vi "Acquire.vi"(0 "Acquisition Unit in (0)":i32, 1 "Replay settings":T19={"Sampling Rate"=0.0, "Samples in replay"=0, "Replay Start Time"=1000.0, "Replay Stop Time"=0.003} {"Replay Stop Time" format="%.3p"; "Replay Start Time" format="%.3p"}, 5 "Acquire Definition":T3={"Acquire Mode"=enum."stop", "Acquisition mode"=enum."Sampled", "Acquirer"=enum."Cleverscope", "Transfer Chans"=enum."Chan A+B", "A max scale"=5.0, "A min scale"=-5.0, "B max scale"=5.0, "B min scale"=-5.0, "A Probe"=enum."x1", "B Probe"=enum."x1", "A Coupling"=enum."DC", "B Coupling"=enum."DC", "A Bandwidth"=1, "B Bandwidth"=1, "Trigger Source"=enum."Chan A", "Trigger Amplitude"=0.0, "A Trigger Amplitude"=0.0, "B Trigger Amplitude"=0.0, "Trigger Filter"=enum."None", "Trig Slope"=FALSE, "Trigger Holdoff"=0.0, "Dig Pattern Rqd"=FALSE, "Dig Pattern"=0, "Ext Trig Threshold"=0.0, "Dig Input Threshold"=0.0, "Start Time"=-0.003, "Stop Time"=0.003, "Pre Trig Time"=0.003, "Port"=enum."Port 1", "Num divisions"=6, "Num seq frames"=1, "Num Buffers"=2, "Sig Gen Freq"=1000.0, "Sig Gen Amp"=1.0, "Sig Gen Offset"=0.0, "Sig Gen Waveform"=enum."sine", "Sig Gen Sweep"=enum."Log", "Sig Gen Func"=enum."Standard", "Sig Gen Freq 2"=1000.0, "Sig Gen Phase"=180.0, "Trig 2 Function"=enum."None", "Min Trigger Period"=1e-08, "Max trigger Period"=0.0001, "Trigger count"=1, "Trig 2 Slope"=FALSE, "Trig 2 Source Chan"=enum."Chan A", "Trig 2 Level"=0.0, "Dig Pattern 2 Rqd"=FALSE, "Dig Pattern 2"=0, "Trigger 2 Source"=enum."Trigger 1 inverted", "Waveform Averages"=0, "Value changed"=0, "Freq Span"=0.0, "Freq Res"=0.0, "Duration"=0.0, "Resolution"=0.0, "Link Port"=enum."Debug", "Ext Sample Clock"=FALSE, "F Spare 2"=FALSE, "F Spare 3"=FALSE, "F Spare 4"=FALSE, "Sampler Resolution"=enum."10 bit", "Intf Source"=enum."USB", "Update Rate"=enum."20 Frame/sec", "Transfer Size"=enum."Normal", "Sig Gen Freq Step"=0.0, "TCP Adr"=0, "TCP port"=0, "CAU Ser Num Hi"=0, "CAU Ser Num Lo"=0, "Function Number"=0.0, "Function Parameter"=0.0, "Function Result"=0.0, "Link Start"=0, "Link Timebase"=0, "Link Timer"=0, "Link Setup"=0, "Spare 1"=0.0, "Spare 2"=0.0, "Spare 3"=0.0, "Spare 4"=0.0} {"Function Result" format="%#.6p"; "Function Parameter" format="%#.6p"; "Function Number" format="%#.6p"; "TCP Adr" format="%08x"; "Sig Gen Freq Step" format="%.2f"; "Sig Gen Phase" format="%.2f"; "Sig Gen Freq 2" format="%.2f"; "Resolution" format="%#.6p"; "Duration" format="%#.6p"; "Freq Res" format="%#.6p"; "Freq Span" format="%#.6p"; "Dig Pattern 2" format="%.0x"; "Trig 2 Level" step=0.001 format="%#.6p"; "Trigger count" step=1; "Max trigger Period" min=1e-08 max=42.9 step=0.01 format="%#.6p"; "Min Trigger Period" min=1e-08 max=42.9 step=0.01 format="%#_6p"; "Sig Gen Offset" format="%.2f"; "Sig Gen Amp" format="%.2f"; "Sig Gen Freq" format="%.2f"; "B Trigger Amplitude" format="%.1p"; "A Trigger Amplitude" format="%.1p"; "B Bandwidth" format="%x"; "A Bandwidth" format="%x"; "B min scale" format="%.2p"; "B max scale" format="%.2p"; "A min scale" format="%.2p"; "A max scale" format="%.2p"; "Trigger Holdoff" format="%.1p"; "Dig Input Threshold" format="%.2f"; "Ext Trig Threshold" format="%.2f"; "Dig Pattern" format="%.0x"; "Pre Trig Time" format="%.3p"; "Start Time" format="%.2p"; "Trigger Amplitude" format="%.1p"; "Stop Time" format="%.2p"}, 11 "error in (no error)":errorcluster, 12 "Stop Refnum":refnum<vi>) -> (3 "T0dt":T2={"T0"=0.0, "dt"=1.0, "n"=0} {"dt" format="%.3p"; "T0" format="%.3p"}, 4 "Acquisition Unit out":i32, 6 "Acquire Defn Out":T3={"Acquire Mode"=enum."stop", "Acquisition mode"=enum."Sampled", "Acquirer"=enum."Cleverscope", "Transfer Chans"=enum."Chan A+B", "A max scale"=5.0, "A min scale"=-5.0, "B max scale"=5.0, "B min scale"=-5.0, "A Probe"=enum."x1", "B Probe"=enum."x1", "A Coupling"=enum."DC", "B Coupling"=enum."DC", "A Bandwidth"=1, "B Bandwidth"=1, "Trigger Source"=enum."Chan A", "Trigger Amplitude"=0.0, "A Trigger Amplitude"=0.0, "B Trigger Amplitude"=0.0, "Trigger Filter"=enum."None", "Trig Slope"=FALSE, "Trigger Holdoff"=0.0, "Dig Pattern Rqd"=FALSE, "Dig Pattern"=0, "Ext Trig Threshold"=0.0, "Dig Input Threshold"=0.0, "Start Time"=-0.003, "Stop Time"=0.003, "Pre Trig Time"=0.003, "Port"=enum."Port 1", "Num divisions"=6, "Num seq frames"=1, "Num Buffers"=2, "Sig Gen Freq"=1000.0, "Sig Gen Amp"=1.0, "Sig Gen Offset"=0.0, "Sig Gen Waveform"=enum."sine", "Sig Gen Sweep"=enum."Log", "Sig Gen Func"=enum."Standard", "Sig Gen Freq 2"=1000.0, "Sig Gen Phase"=180.0, "Trig 2 Function"=enum."None", "Min Trigger Period"=1e-08, "Max trigger Period"=0.0001, "Trigger count"=1, "Trig 2 Slope"=FALSE, "Trig 2 Source Chan"=enum."Chan A", "Trig 2 Level"=0.0, "Dig Pattern 2 Rqd"=FALSE, "Dig Pattern 2"=0, "Trigger 2 Source"=enum."Trigger 1 inverted", "Waveform Averages"=0, "Value changed"=0, "Freq Span"=0.0, "Freq Res"=0.0, "Duration"=0.0, "Resolution"=0.0, "Link Port"=enum."Debug", "Ext Sample Clock"=FALSE, "F Spare 2"=FALSE, "F Spare 3"=FALSE, "F Spare 4"=FALSE, "Sampler Resolution"=enum."10 bit", "Intf Source"=enum."USB", "Update Rate"=enum."20 Frame/sec", "Transfer Size"=enum."Normal", "Sig Gen Freq Step"=0.0, "TCP Adr"=0, "TCP port"=0, "CAU Ser Num Hi"=0, "CAU Ser Num Lo"=0, "Function Number"=0.0, "Function Parameter"=0.0, "Function Result"=0.0, "Link Start"=0, "Link Timebase"=0, "Link Timer"=0, "Link Setup"=0, "Spare 1"=0.0, "Spare 2"=0.0, "Spare 3"=0.0, "Spare 4"=0.0} {"Function Result" format="%#.6p"; "Function Parameter" format="%#.6p"; "Function Number" format="%#.6p"; "TCP Adr" format="%08x"; "Sig Gen Freq Step" format="%.2f"; "Sig Gen Phase" format="%.2f"; "Sig Gen Freq 2" format="%.2f"; "Resolution" format="%#.6p"; "Duration" format="%#.6p"; "Freq Res" format="%#.6p"; "Freq Span" format="%#.6p"; "Dig Pattern 2" format="%.0x"; "Trig 2 Level" step=0.001 format="%#.6p"; "Trigger count" step=1; "Max trigger Period" min=1e-08 max=42.9 step=0.01 format="%#.6p"; "Min Trigger Period" min=1e-08 max=42.9 step=0.01 format="%#_6p"; "Sig Gen Offset" format="%.2f"; "Sig Gen Amp" format="%.2f"; "Sig Gen Freq" format="%.2f"; "B Trigger Amplitude" format="%.1p"; "A Trigger Amplitude" format="%.1p"; "B Bandwidth" format="%x"; "A Bandwidth" format="%x"; "B min scale" format="%.2p"; "B max scale" format="%.2p"; "A min scale" format="%.2p"; "A max scale" format="%.2p"; "Trigger Holdoff" format="%.1p"; "Dig Input Threshold" format="%.2f"; "Ext Trig Threshold" format="%.2f"; "Dig Pattern" format="%.0x"; "Pre Trig Time" format="%.3p"; "Start Time" format="%.2p"; "Trigger Amplitude" format="%.1p"; "Stop Time" format="%.2p"}, 8 "Chan AB Data":cluster{"Chan A Data":T1[], "Chan B Data":T1[]} {"Chan A Data" format="%_6p"; "Chan B Data" format="%_6p"}, 14 "Waveform":waveform(sgl)[](array[waveform]), 15 "error out":errorcluster)   [LabVIEW 2009]
uses:
  libraries/Cscope control driver.llb/Acquire Event type.ctl
  libraries/Cscope control driver.llb/Acquire capture type.ctl
  libraries/Cscope control driver.llb/Acquire capture method.ctl
  libraries/Cscope control driver.llb/Acquirer type.ctl
  libraries/Cscope control driver.llb/Input Range.ctl
  libraries/Cscope control driver.llb/Input Coupling.ctl
  libraries/Cscope control driver.llb/Input Bandwidth.ctl
  libraries/Cscope control driver.llb/USB channel.ctl
  libraries/Cscope control driver.llb/Trigger Filter.ctl
  libraries/Cscope control driver.llb/Cscope waveform type.ctl
  libraries/Cscope control driver.llb/Trigger Period.ctl
  libraries/Cscope control driver.llb/Trigger channel.ctl
  libraries/Cscope control driver.llb/Link port types.ctl
  libraries/Cscope control driver.llb/Acquirer resolution.ctl
  libraries/Cscope control driver.llb/Intf source.ctl
  libraries/Cscope control driver.llb/Acquire transfer size.ctl
  typedefs/Cscope/ReplaySettings.ctl
  libraries/Cscope control driver.llb/QSig_T0dt.ctl
  libraries/Cscope control driver.llb/Cscope real.ctl
  libraries/Cscope control driver.llb/Cscope control command type.ctl
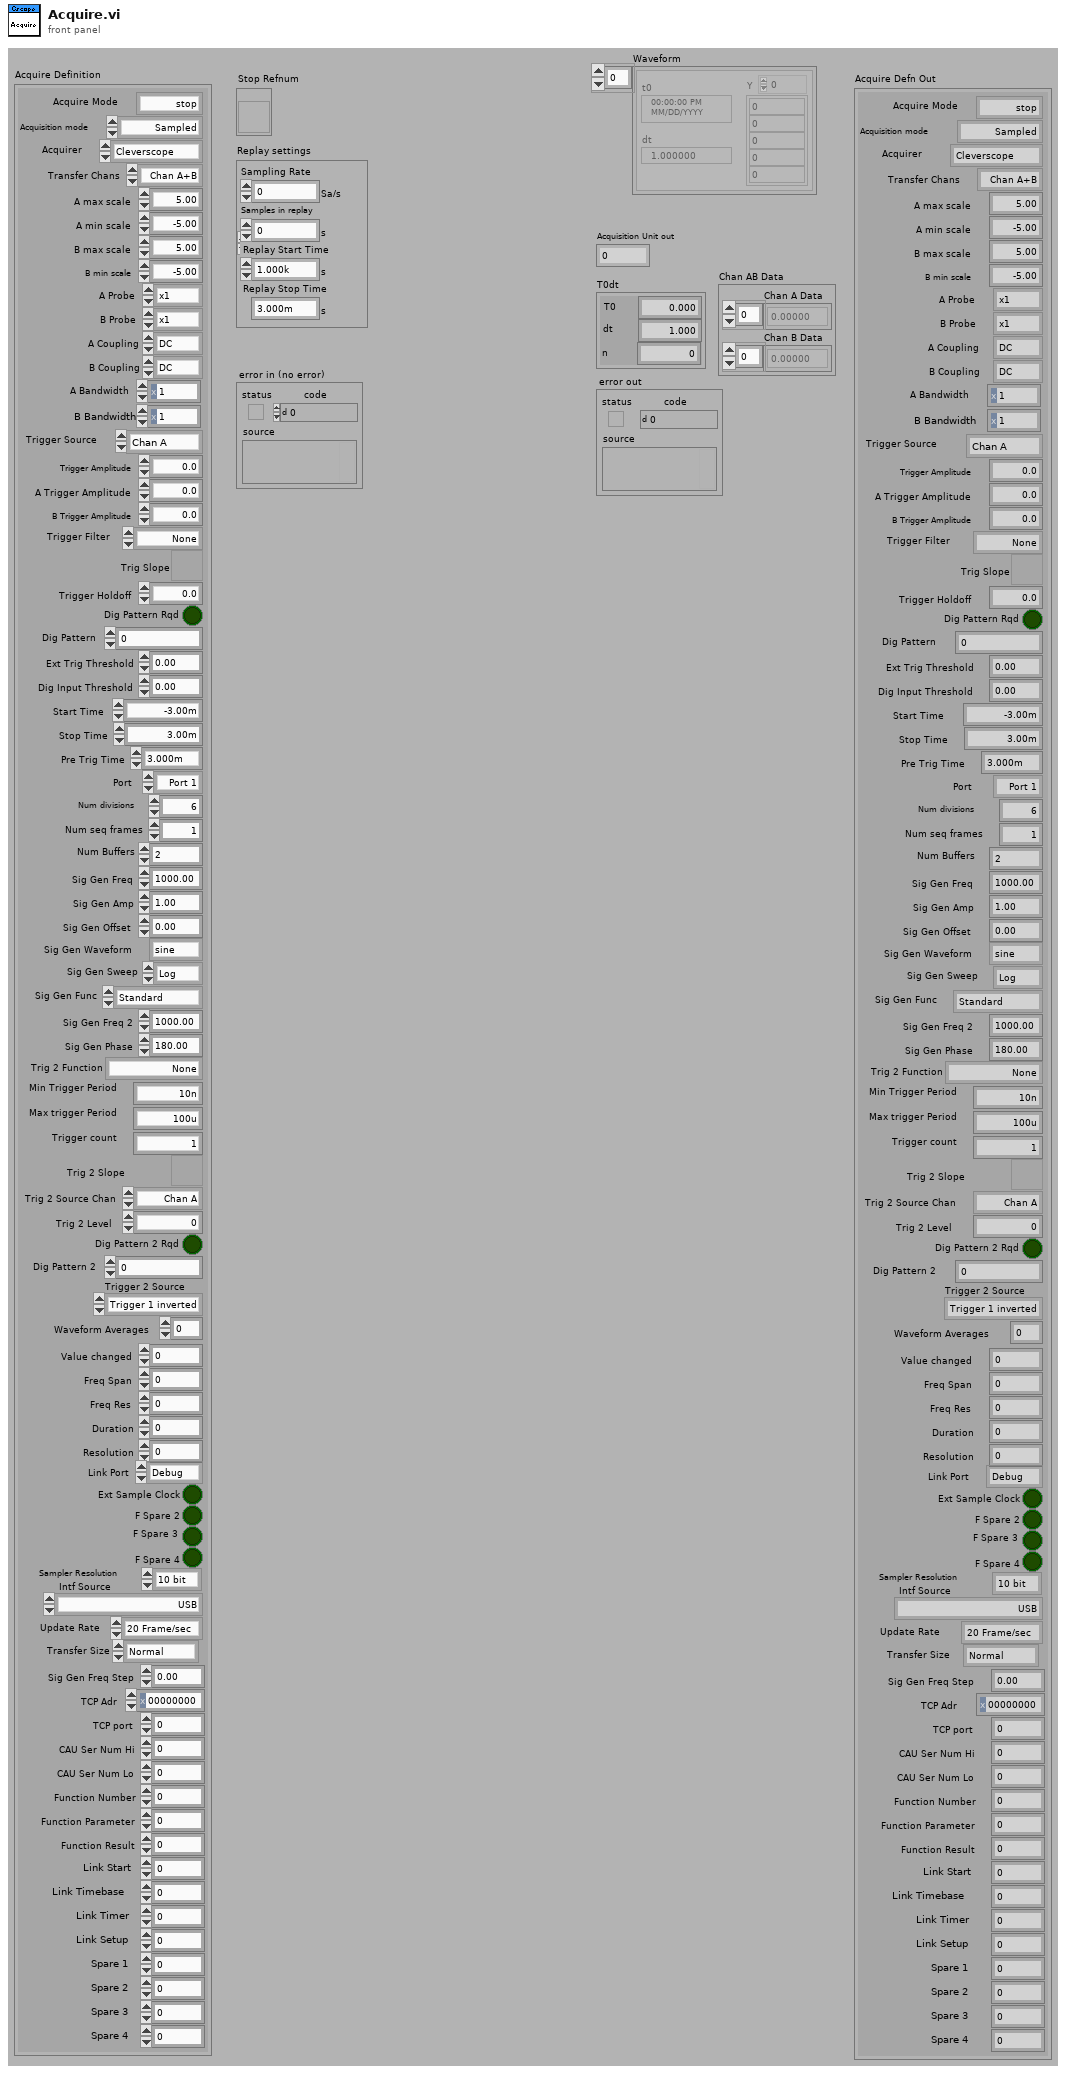
[diagram p1: front panel]
types:
  T1 = typedef "Cscope real.ctl" = sgl
  T2 = typedef "QSig_T0dt.ctl" = cluster{"T0":dbl, "dt":dbl, "n":i32}
  T3 = typedef "Acquire Event type.ctl" = cluster{"Acquire Mode":T4, "Acquisition mode":T5, "Acquirer":T6, "Transfer Chans":enum16{"Chan A", "Chan B", "Chan A+B"}, "A max scale":dbl, "A min scale":dbl, "B max scale":dbl, "B min scale":dbl, "A Probe":T7, "B Probe":T7, "A Coupling":T8, "B Coupling":T8, "A Bandwidth":T9, "B Bandwidth":T9, "Trigger Source":T10, "Trigger Amplitude":dbl, "A Trigger Amplitude":dbl, "B Trigger Amplitude":dbl, "Trigger Filter":T11, "Trig Slope":bool, "Trigger Holdoff":dbl, "Dig Pattern Rqd":bool, "Dig Pattern":u32, "Ext Trig Threshold":dbl, "Dig Input Threshold":dbl, "Start Time":dbl, "Stop Time":dbl, "Pre Trig Time":dbl, "Port":enum16{"Port 1", "Port 2", "Port 3", "Port 4", "Port 5", "Port 6"}, "Num divisions":i16, "Num seq frames":i16, "Num Buffers":i32, "Sig Gen Freq":dbl, "Sig Gen Amp":dbl, "Sig Gen Offset":dbl, "Sig Gen Waveform":T12, "Sig Gen Sweep":enum16{"Linear", "Log"}, "Sig Gen Func":enum16{"Standard", "Auto advance", "Freq mod In8", "Phase mod In8"}, "Sig Gen Freq 2":dbl, "Sig Gen Phase":dbl, "Trig 2 Function":T13, "Min Trigger Period":dbl, "Max trigger Period":dbl, "Trigger count":u32, "Trig 2 Slope":bool, "Trig 2 Source Chan":T14, "Trig 2 Level":dbl, "Dig Pattern 2 Rqd":bool, "Dig Pattern 2":u32, "Trigger 2 Source":enum16{"Trigger 1 inverted", "Trig 2 Defn"}, "Waveform Averages":i32, "Value changed":i32, "Freq Span":dbl, "Freq Res":dbl, "Duration":dbl, "Resolution":dbl, "Link Port":T15, "Ext Sample Clock":bool, "F Spare 2":bool, "F Spare 3":bool, "F Spare 4":bool, "Sampler Resolution":T16, "Intf Source":T17, "Update Rate":enum16{"20 Frame/sec", "10 Frame/sec", "5 Frame/sec"}, "Transfer Size":T18, "Sig Gen Freq Step":dbl, "TCP Adr":u32, "TCP port":u32, "CAU Ser Num Hi":u32, "CAU Ser Num Lo":u32, "Function Number":dbl, "Function Parameter":dbl, "Function Result":dbl, "Link Start":u32, "Link Timebase":u32, "Link Timer":u32, "Link Setup":u32, "Spare 1":dbl, "Spare 2":dbl, "Spare 3":dbl, "Spare 4":dbl}
  T4 = typedef "Acquire capture type.ctl" = enum16{"single", "automatic", "triggered", "stop", "single stop", "replay"}
  T5 = typedef "Acquire capture method.ctl" = enum16{"Sampled", "Peak Captured", "Filtered", "Repetitive", "Waveform avg"}
  T6 = typedef "Acquirer type.ctl" = enum16{"Internal Sig Gen", "APC 901", "APC 901A", "Sound Card", "Cleverscope"}
  T7 = typedef "Input Range.ctl" = enum16{"x1", "x10", "x100", "x1K", "x20", "x50", "x200"}
  T8 = typedef "Input Coupling.ctl" = enum16{"AC", "DC"}
  T9 = typedef "Input Bandwidth.ctl" = u16
  T10 = typedef "USB channel.ctl" = enum32{"Chan A", "Chan B", "Ext Trigger", "Dig Trig", "Link Input", "chan_5", "chan_6", "chan_7", "chan_8", "chan_9", "chan_10", "chan_11", "chan_12", "chan_13", "chan_14", "chan_15"}
  T11 = typedef "Trigger Filter.ctl" = enum16{"None", "Low Pass", "Hi Pass", "Noise"}
  T12 = typedef "Cscope waveform type.ctl" = enum16{"sine", "triangle", "square", "DC", "OFF"}
  T13 = typedef "Trigger Period.ctl" = enum16{"None", "Trig 1~2 < min", "min<T1~2 < max", "Trig 1~2 > max", "Count Trig 1", "Count Trig 2"}
  T14 = typedef "Trigger channel.ctl" = enum32{"Chan A", "Chan B", "Ext Trigger", "Dig Trig", "Link Input"}
  T15 = typedef "Link port types.ctl" = enum8{"Debug", "Link Out", "Disabled", "Slave", "Master", "Uart", "SPI", "I2C", "Digital", "Sig Gen"}
  T16 = typedef "Acquirer resolution.ctl" = enum16{"10 bit", "12 Bit", "14 bit"}
  T17 = typedef "Intf source.ctl" = enum16{"USB", "Ethernet - Find by IP address", "Ethernet - Find first IP address", "Ethernet - Find by serial number"}
  T18 = typedef "Acquire transfer size.ctl" = enum16{"Normal", "100% Buffer", "50% Buffer", "10% Buffer", "5% Buffer", "2% Buffer", "Sequence"}
  T19 = typedef "ReplaySettings.ctl" = cluster{"Sampling Rate":dbl, "Samples in replay":u32, "Replay Start Time":dbl, "Replay Stop Time":dbl}
  T20 = typedef "Cscope control command type.ctl" = enum16{"Initialize", "Acquire", "Replay", "Wait for samples", "Update", "Close", "Status", "Function", "Get Frame", "Finish", "Function Result", "Check Got Samples", "Get Chan A", "Get Chan B", "Get Dig"}
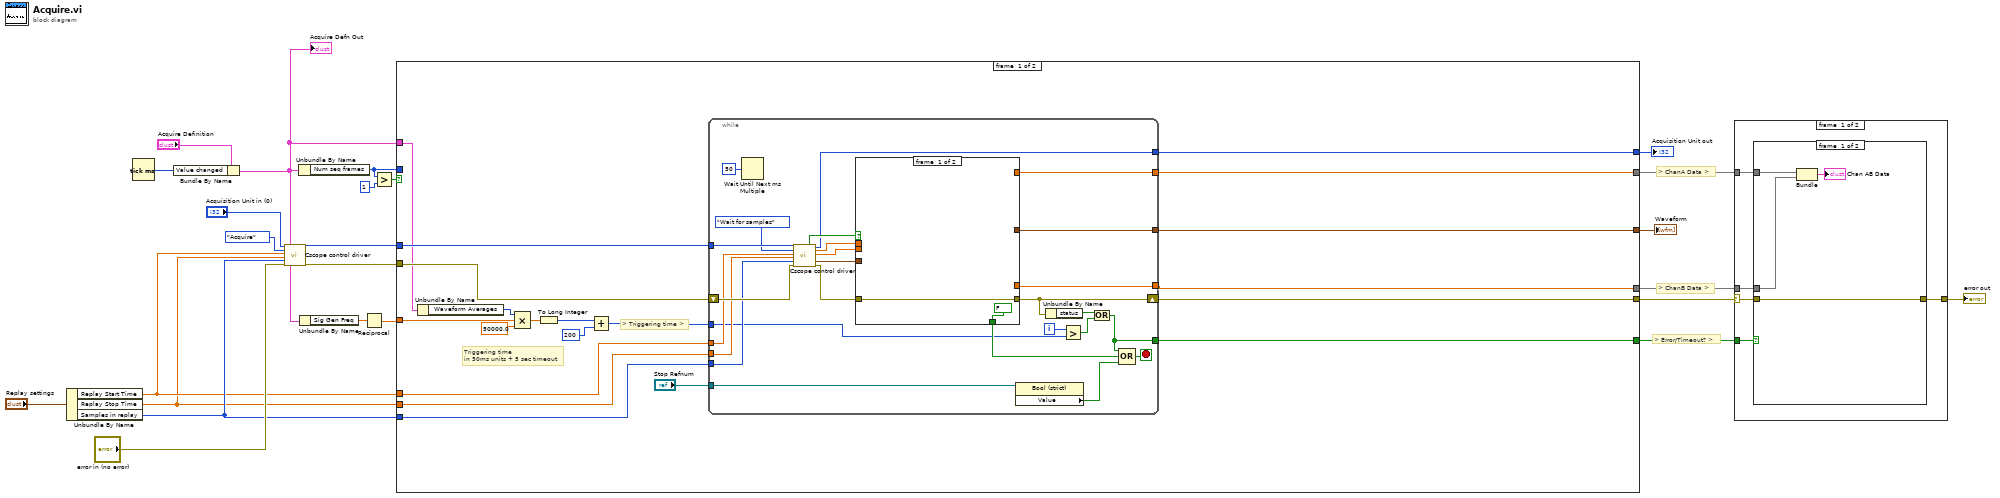
[diagram p0: block diagram]
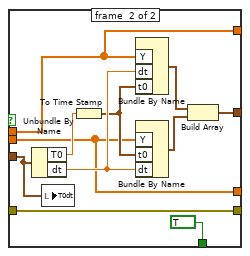
[diagram p2: hidden frame]
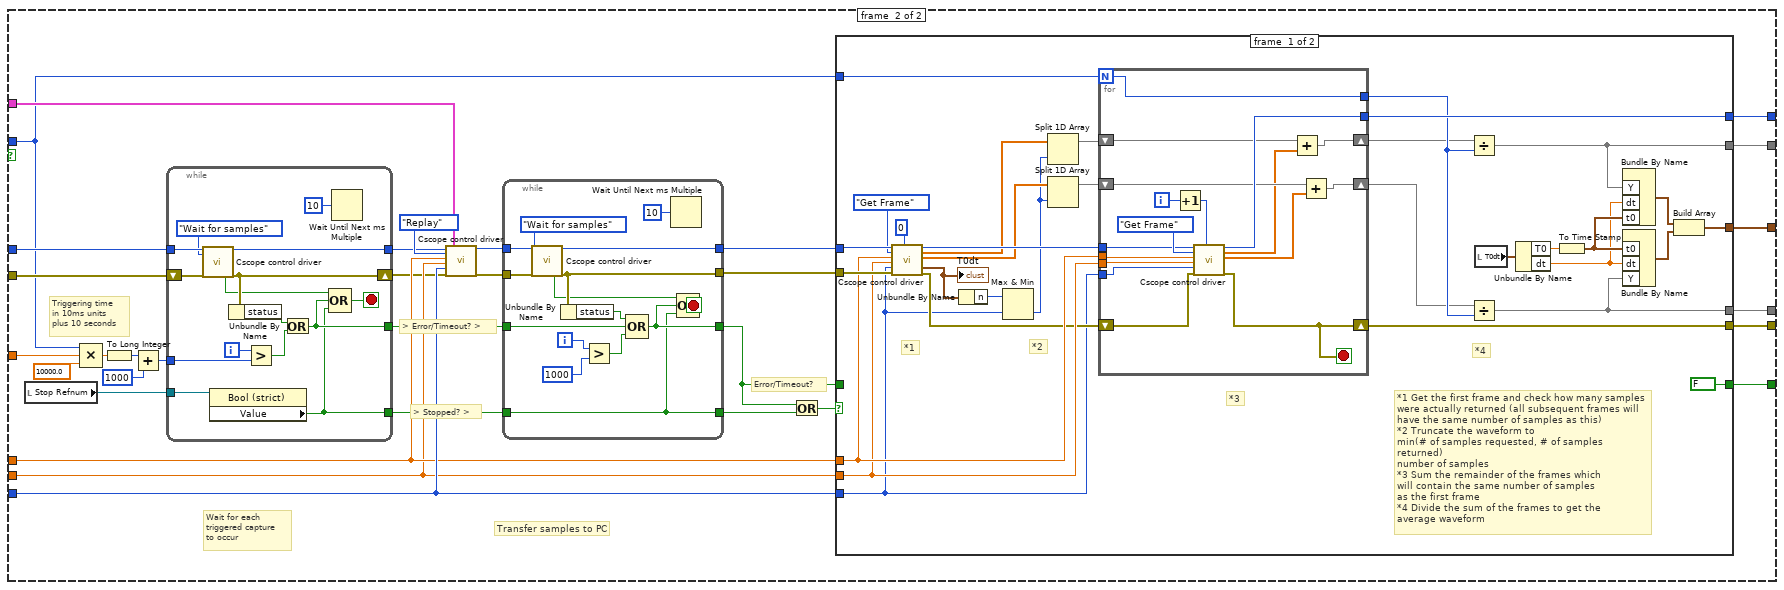
[diagram p3: hidden frame]
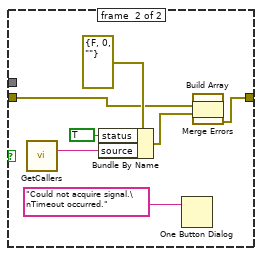
[diagram p5: hidden frame]
diagram:
  # "> Error/Timeout? >"
  # "> ChanB Data >"
  # "> ChanA Data >"
  n1 = Unbundle By Name("Replay settings") -> ("Replay Start Time"=w15:dbl, "Replay Stop Time"=w14:dbl, "Samples in replay"=w20:u32)
  n2 = Tick Count (ms)() -> (millisecond timer value=w19:u32)
  n3 = Bundle By Name(cluster="Acquire Definition", "Value changed"=w19) -> (w6:T3)
  "Acquire Defn Out" <- w6
  n4 = call "Cscope control driver.vi"("Acquisition Unit in"="Acquisition Unit in (0)", "Command"=Cscope_control_command_type."Acquire", "Replay Start Time"=w15, "Replay Stop Time"=w14, "Samples in replay"=w20, "error in"="error in (no error)", "Acquire Definition"=w6) -> ("Acquisition Unit out"=w8:i32, "error out"=w9:errorcluster)  [unwired: 1 in, 10 out]
  n5 = Unbundle By Name(w6) -> ("Num seq frames"=w7:i16)
  n6 = Unbundle By Name(w6) -> ("Sig Gen Freq"=w5:dbl)
  n7 = Reciprocal(x=w5) -> (1/x=w4:dbl)
  n8 = Greater?(x=w7, y=i16 1) -> (0:w10:bool)
  n9 = case shown="True" w10 {
    tunnel: w8 -> [w44 w101]
    tunnel: w9 -> [w43 w102]
    tunnel: w20 -> [w31 w110]
    tunnel: [w41 w109] -> w18
    tunnel: [w40 w104] -> w17
    tunnel: w15 -> [w39 w108]
    tunnel: w14 -> [w38 w107]
    tunnel: w6 -> [w37 w106]
    tunnel: [w42 w105] -> w11
    tunnel: w7 -> [_ w98]
    tunnel: w4 -> [w35 w97]
    tunnel: [w29 w87] -> w3
    tunnel: [w28 w91] -> w2
    tunnel: [w30 w90] -> w1
    frame #0 {
      # "> Triggering time >"
      # "Triggering time\nin 50ms units + 5 sec timeout"
      n10 = Unbundle By Name(w37) -> ("Waveform Averages"=w36:i32)
      n11 = Compound Arithmetic op=MULTIPLY(w36, w35, 50000.0 ("value")) -> (w33:dbl)
      n12 = To Long Integer(number=w33) -> (32bit integer=w26:i32)
      n13 = Add(x=w26, y=200) -> (x+y=w25:i32)
      n14 = while {
        tunnel: w44 -> [w70]
        tunnel: [w63] -> w42
        shift-right: [w57] -> w41
        shift-left: w43 -> [w69]
        tunnel: [w54] -> w40
        tunnel: [w53] -> w30
        tunnel: w39 -> [w52]
        tunnel: w38 -> [w51]
        tunnel: w25 -> [w45]
        tunnel: "Stop Refnum" -> [w50]
        tunnel: w31 -> [w49]
        tunnel: [w48] -> w29
        tunnel: [w47] -> w28
        i -> [w60]
        stop <- w59 stop-if-true
        n15 = Wait Until Next ms Multiple(millisecond multiple=u32 50) -> ()  [unwired: 1 out]
        n16 = call "Cscope control driver.vi"("Acquisition Unit in"=w70, "Command"=Cscope_control_command_type."Wait for samples", "Replay Start Time"=w52, "Replay Stop Time"=w51, "Samples in replay"=w49, "error in"=w69) -> ("Got Samples"=w64:bool, "Acquisition Unit out"=w63:i32, "Chan A Data"=w66:T1[], "Chan B Data"=w68:T1[], "T0dt"=w65:T2, "error out"=w61:errorcluster)  [unwired: 2 in, 6 out]
        n17 = case shown="True" w64 {
          tunnel: w68 -> [_ w74]
          tunnel: [_ w80] -> w53
          tunnel: w66 -> [_ w75]
          tunnel: w65 -> [_ w73]
          tunnel: [FALSE TRUE] -> w58
          tunnel: w61 -> [w72 w78]
          tunnel: [w72 w78] -> w57
          tunnel: [_ w75] -> w48
          tunnel: [_ w74] -> w47
          frame #0 {
          }
          frame #1 {
            n18 = Unbundle By Name(w73) -> ("T0"=w82:dbl, "dt"=w83:dbl)
            n19 = local write "T0dt"(w73) -> ()
            n20 = To Time Stamp(1:w82) -> (0:w81:timestamp)
            n21 = Bundle By Name("Y"=w75, "dt"=w83, "t0"=w81) -> (w77:waveform(sgl))  [unwired: 1 out]
            n22 = Bundle By Name("Y"=w74, "t0"=w81, "dt"=w83) -> (w76:waveform(sgl))  [unwired: 1 out]
            n23 = Build Array(w77, w76) -> (w80:waveform(sgl)[])
          }
        }
        n24 = property class="Bool (strict)"(reference=w50) -> ("Value"=w46:bool)  [unwired: 1 in, 2 out]
        n25 = Unbundle By Name(w57) -> ("status"=w56:bool)
        n26 = Greater?(x=w60, y=w45) -> (0:w55:bool)
        n27 = Or(x=w56, y=w55) -> (x .or. y?=w54:bool)
        n28 = Compound Arithmetic op=OR(w54, w58, w46) -> (w59:bool)
      }
    }
    frame #1 {
      # "> Stopped? >"
      # "Error/Timeout?"
      # "> Error/Timeout? >"
      # "Wait for each\ntriggered capture\nto occur"
      # "Transfer samples to PC"
      # "Triggering time\nin 10ms units\nplus 10 seconds"
      n29 = local read "Stop Refnum"() -> (w94:refnum<vi>)
      n30 = Compound Arithmetic op=MULTIPLY(w98, w97, 10000.0 ("value")) -> (w95:dbl)
      n31 = To Long Integer(number=w95) -> (32bit integer=w86:i32)
      n32 = Add(x=w86, y=1000) -> (x+y=w84:i32)
      n33 = while {
        tunnel: w101 -> [w180]
        tunnel: [w179] -> w99
        shift-right: [w177] -> w100
        shift-left: w102 -> [w181]
        tunnel: [w170] -> w103
        tunnel: w94 -> [w172]
        tunnel: [w169] -> w93
        tunnel: w84 -> [w168]
        i -> [w176]
        stop <- w171 stop-if-true
        n34 = call "Cscope control driver.vi"("Acquisition Unit in"=w180, "Command"=Cscope_control_command_type."Wait for samples", "error in"=w181) -> ("Got Samples"=w175:bool, "Acquisition Unit out"=w179:i32, "error out"=w177:errorcluster)  [unwired: 5 in, 9 out]
        n35 = property class="Bool (strict)"(reference=w172) -> ("Value"=w169:bool)  [unwired: 1 in, 2 out]
        n36 = Unbundle By Name(w177) -> ("status"=w174:bool)
        n37 = Greater?(x=w176, y=w168) -> (0:w173:bool)
        n38 = Or(x=w174, y=w173) -> (x .or. y?=w170:bool)
        n39 = Compound Arithmetic op=OR(w175, w170, w169) -> (w171:bool)
        n40 = Wait Until Next ms Multiple(millisecond multiple=u32 10) -> ()  [unwired: 1 out]
      }
      n41 = call "Cscope control driver.vi"("Acquisition Unit in"=w99, "Command"=Cscope_control_command_type."Replay", "Replay Start Time"=w108, "Replay Stop Time"=w107, "Samples in replay"=w110, "error in"=w100, "Acquire Definition"=w106) -> ("Acquisition Unit out"=w113:i32, "error out"=w115:errorcluster)  [unwired: 1 in, 10 out]
      n42 = while {
        tunnel: w115 -> [w197]
        tunnel: w113 -> [w196]
        tunnel: [w195] -> w112
        tunnel: [w194] -> w111
        tunnel: w103 -> [w187]
        tunnel: [w184] -> w89
        tunnel: w93 -> [w183]
        tunnel: [w183] -> w88
        i -> [w190]
        stop <- w191 stop-if-true
        n43 = call "Cscope control driver.vi"("Acquisition Unit in"=w196, "Command"=Cscope_control_command_type."Wait for samples", "error in"=w197) -> ("Got Samples"=w186:bool, "Acquisition Unit out"=w194:i32, "error out"=w195:errorcluster)  [unwired: 5 in, 9 out]
        n44 = Unbundle By Name(w195) -> ("status"=w185:bool)
        n45 = Greater?(x=w190, y=1000) -> (0:w188:bool)
        n46 = Compound Arithmetic op=OR(w185, w187, w188) -> (w184:bool)
        n47 = Wait Until Next ms Multiple(millisecond multiple=u32 10) -> ()  [unwired: 1 out]
        n48 = Compound Arithmetic op=OR(w186, w184, w183) -> (w191:bool)
      }
      n49 = Or(x=w89, y=w88) -> (x .or. y?=w92:bool)
      n50 = case shown="False" w92 {
        tunnel: w112 -> [w131 w166]
        tunnel: w111 -> [w132 w167]
        tunnel: w110 -> [w116 _]
        tunnel: [w147 w166] -> w109
        tunnel: w108 -> [w129 _]
        tunnel: w107 -> [w128 _]
        tunnel: [w146 w167] -> w105
        tunnel: [FALSE w165] -> w104
        tunnel: w98 -> [w145 _]
        tunnel: w89 -> [_ w165]
        tunnel: [w138 _] -> w91
        tunnel: [w144 _] -> w90
        tunnel: [w135 _] -> w87
        frame #0 {
          # "*4"
          # "*3"
          # "*1 Get the first frame and check how many samples \nwere actually returned (all subsequent frames will\nhave the same number of samples as this)\n*2 Truncate the waveform to \nmin(# of samples requested, # of samples returned)\nnumber of samples\n*3 Sum the remainder of the frames which\nwill contain the same number of samples\nas the first frame\n*4 Divide the sum of the frames to get the\naverage waveform"
          # "*2"
          # "*1"
          n51 = call "Cscope control driver.vi"("Acquisition Unit in"=w132, "Command"=Cscope_control_command_type."Get Frame", "Replay Start Time"=w129, "Replay Stop Time"=w128, "Samples in replay"=w116, "error in"=w131, "Frame Number"=0) -> ("Acquisition Unit out"=w133:i32, "Chan A Data"=w123:T1[], "Chan B Data"=w121:T1[], "T0dt"=w125:T2, "error out"=w127:errorcluster)  [unwired: 1 in, 7 out]
          "T0dt" <- w125
          n52 = Unbundle By Name(w125) -> ("n"=w124:i32)
          n53 = Max & Min(x=w124, y=w116) -> (min(x,y)=w119:u32)  [unwired: 1 out]
          n54 = Split 1D Array(array=w123, index=w119) -> (first subarray=w122:T1[])  [unwired: 1 out]
          n55 = Split 1D Array(array=w121, index=w119) -> (first subarray=w120:T1[])  [unwired: 1 out]
          n56 = for {
            N: w145 -> [w155]
            tunnel: [w164] -> w146
            tunnel: w129 -> [w162]
            tunnel: w128 -> [w161]
            tunnel: w133 -> [w159]
            shift-right: [w158] -> w147
            shift-left: w127 -> [w160]
            shift-right: [w157] -> w117
            shift-left: w122 -> [w156]
            tunnel: [w155] -> w142
            shift-right: [w154] -> w118
            shift-left: w120 -> [w153]
            tunnel: w116 -> [w148]
            i -> [w152]
            stop <- w158 stop-if-true
            n57 = Increment(x=w152) -> (x+1=w151:i32)
            n58 = call "Cscope control driver.vi"("Acquisition Unit in"=w159, "Command"=Cscope_control_command_type."Get Frame", "Replay Start Time"=w162, "Replay Stop Time"=w161, "Samples in replay"=w148, "error in"=w160, "Frame Number"=w151) -> ("Acquisition Unit out"=w164:i32, "Chan A Data"=w149:T1[], "Chan B Data"=w150:T1[], "error out"=w158:errorcluster)  [unwired: 1 in, 8 out]
            n59 = Add(x=w156, y=w149) -> (x+y=w157:T1[])
            n60 = Add(x=w153, y=w150) -> (x+y=w154:T1[])
          }
          n61 = Divide(x=w117, y=w142) -> (x/y=w135:T1[])
          n62 = Divide(x=w118, y=w142) -> (x/y=w138:T1[])
          n63 = local read "T0dt"() -> (w134:T2)
          n64 = Unbundle By Name(w134) -> ("T0"=w141:dbl, "dt"=w139:dbl)
          n65 = To Time Stamp(1:w141) -> (0:w140:timestamp)
          n66 = Bundle By Name("Y"=w135, "dt"=w139, "t0"=w140) -> (w137:waveform(sgl))  [unwired: 1 out]
          n67 = Bundle By Name("t0"=w140, "dt"=w139, "Y"=w138) -> (w136:waveform(sgl))  [unwired: 1 out]
          n68 = Build Array(w137, w136) -> (w144:waveform(sgl)[])
        }
        frame #1 {
        }
      }
    }
  }
  "Acquisition Unit out" <- w11
  "Waveform" <- w1
  n69 = case shown="No Error" w18 {
    selector: w18 -> [w200 w215]
    tunnel: w17 -> [w202 _]
    tunnel: [w201 w215] -> w16
    tunnel: w3 -> [w199 _]
    tunnel: w2 -> [w198 _]
    frame #0 {
      n70 = case shown="False" w202 {
        tunnel: [w206 w214] -> w201
        tunnel: w200 -> [w206 w209]
        tunnel: w199 -> [w205 _]
        tunnel: w198 -> [w204 _]
        frame #0 {
          n71 = Bundle("Chan A Data"=w205, "Chan B Data"=w204) -> (→"Chan AB Data":cluster{"Chan A Data":T1[], "Chan B Data":T1[]})  [unwired: 1 in]
        }
        frame #1 {
          n72 = call "GetCallers.vi"() -> ("Caller String"=w211:string)  [unwired: 15 in]
          n73 = Bundle By Name(cluster=errorcluster {"status"=FALSE, "code"=0, "source"=""} ("error in 2 (no error)"), "status"=TRUE, "source"=w211) -> (w208:errorcluster)
          n74 = One Button Dialog(message="Could not acquire signal.\nTimeout occurred.") -> ()  [unwired: 1 in, 1 out]
          n75 = Build Array(w209, w208) -> (w207:errorcluster[])
          n76 = call <vilib>:"Merge Errors.vi"("error array in"=w207) -> ("error out"=w214:errorcluster)  [unwired: 6 in]
        }
      }
    }
    frame #1 {
    }
  }
  "error out" <- w16
